vi "71_DC Motor_PID_final.vi"() -> ()   [LabVIEW 2018]
uses:
  <userlib>/KNR OS 4.0 LabVIEW Toolkit/Type Definition/Resource.ctl
  <userlib>/KNR OS 4.0 LabVIEW Toolkit/Type Definition/DC Motor Port.ctl
panel:
  out "Velocity (cm/sec) 2":dbl
  out "Speed (+-100%) 2":dbl
  out "Speed (+-100%)":dbl
  in  "Desire Velosity (cm/sec)":dbl(slide) scale=-200.0..200.0
  in  "IP":string(combo)="172.22.11.2"
  in  "Resource":T1=enum."KNRm_DDDD"
  in  "stop":bool
  out "Velocity (cm/sec)":dbl
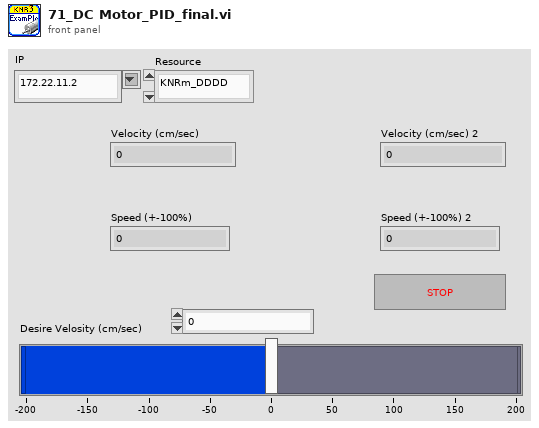
[diagram p1: front panel]
types:
  T1 = typedef "Resource.ctl" = enum16{"KNRm_DDRC", "KNRm_DDDD", "KNRm_DDDR", "KNRm_DDDC", "KNR", "KNRm_neww"}
  T2 = typedef "KNR3 Reference.ctl" = cluster{"FPGA Session":refnum<class "FPGA Interface Base.lvclass">, "Resource":T1}
  T3 = typedef "DC Motor Port.ctl" = u16
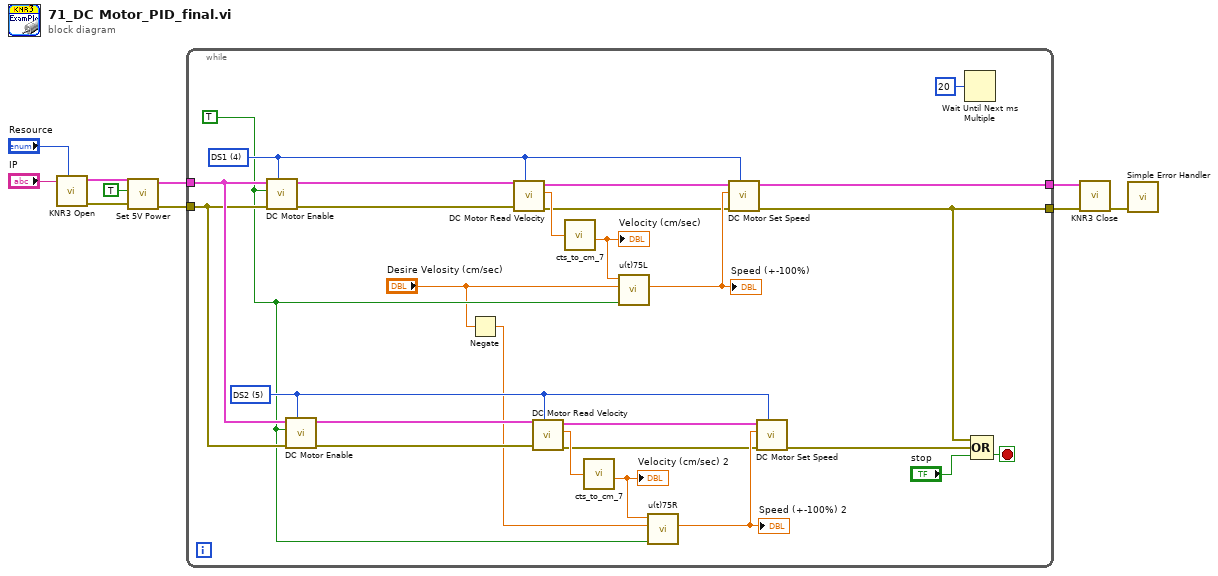
[diagram p0: block diagram]
diagram:
  n1 = call <userlib>:"KNR3 Open.vi"("Resource"="Resource", "IP"="IP") -> ("error out"=w4:errorcluster, "KNR out"=w6:T2)  [unwired: 8 in]
  n2 = call <userlib>:"Set 5V Power.vi"("error in (no error)"=w4, "5V Power(T)"=TRUE ("5V Power"), "KNR in"=w6) -> ("error out"=w8:errorcluster, "KNR out"=w9:T2)  [unwired: 7 in]
  n3 = while {
    tunnel: w9 -> [w24]
    tunnel: w8 -> [w23]
    tunnel: [w30] -> w2
    tunnel: [w22] -> w1
    stop <- w36 stop-if-true
    w20 = TRUE ("Enable Motor")
    w28 = T3 5 items=["DS1"=4, "DS2"=5, "DS3"=6, "DS4"=7] ("Port 2")
    w31 = T3 4 items=["DS1"=4, "DS2"=5, "DS3"=6, "DS4"=7] ("Port")
    n4 = call <userlib>:"DC Motor Enable.vi"("Port (DS1)"=w31, "error in (no error)"=w23, "Enable Motor(F)"=w20, "KNR in"=w24) -> ("error out"=w33:errorcluster, "KNR out"=w34:T2)  [unwired: 6 in]
    n5 = call <userlib>:"DC Motor Enable.vi"("Port (DS1)"=w28, "error in (no error)"=w23, "Enable Motor(F)"=w20, "KNR in"=w24) -> ("error out"=w26:errorcluster, "KNR out"=w25:T2)  [unwired: 6 in]
    n6 = Negate(x="Desire Velosity (cm/sec)") -> (-x=w11:dbl)
    n7 = call <userlib>:"DC Motor Read Velocity.vi"("Port (DS1)"=w31, "error in (no error)"=w33, "KNR in"=w34) -> ("error out"=w17:errorcluster, "Velocity (cts/sec)"=w32:dbl, "KNR out"=w18:T2)  [unwired: 6 in]
    n8 = call <userlib>:"DC Motor Read Velocity.vi"("Port (DS1)"=w28, "error in (no error)"=w26, "KNR in"=w25) -> ("error out"=w15:errorcluster, "Velocity (cts/sec)"=w27:dbl, "KNR out"=w16:T2)  [unwired: 6 in]
    n9 = call "cts_to_cm_7.vi"("cts"=w32) -> ("cm"=w13:dbl)
    "Velocity (cm/sec)" <- w13
    n10 = call "cts_to_cm_7.vi"("cts"=w27) -> ("cm"=w12:dbl)
    "Velocity (cm/sec) 2" <- w12
    n11 = call "u(t)75L.vi"("Velocity"=w13, "Desire Velosity"="Desire Velosity (cm/sec)", "enable"=w20) -> ("u(t)"=w29:dbl)  [unwired: 7 in]
    "Speed (+-100%)" <- w29
    n12 = call "u(t)75R.vi"("Velocity"=w12, "Desire Velosity"=w11, "enable"=w20) -> ("u(t)"=w19:dbl)  [unwired: 7 in]
    "Speed (+-100%) 2" <- w19
    n13 = call <userlib>:"DC Motor Set Speed.vi"("Port (DS1)"=w31, "error in (no error)"=w17, "Speed (+-100%)"=w29, "KNR in"=w18) -> ("error out"=w22:errorcluster, "KNR out"=w30:T2)  [unwired: 6 in]
    n14 = call <userlib>:"DC Motor Set Speed.vi"("Port (DS1)"=w28, "error in (no error)"=w15, "Speed (+-100%)"=w19, "KNR in"=w16) -> ("error out"=w21:errorcluster)  [unwired: 6 in, 1 out]
    n15 = Wait Until Next ms Multiple(millisecond multiple=u32 20) -> ()  [unwired: 1 out]
    n16 = Compound Arithmetic op=OR(w22, w21, "stop") -> (w36:bool)
  }
  n17 = call <userlib>:"KNR3 Close.vi"("error in (no error)"=w1, "KNR in"=w2) -> ("error out"=w7:errorcluster)  [unwired: 9 in]
  n18 = call <vilib>:"Simple Error Handler.vi"("error in (no error)"=w7) -> ()  [unwired: 4 in, 5 out]
